vi "DataSender.vi"() -> ()   [LabVIEW 2013]
uses:
  <vilib>/userdefined/High Color/IMAQdx.ctl
  <vilib>/DAQmx/read.llb/DAQmx Read (Analog 2D DBL NChan NSamp).vi
  <vilib>/DAQmx/miscellaneous.llb/DAQmx Fill In Error Info.vi
  <vilib>/vision/driver/NI_Vision_Acquisition_Software.lvlib
panel:
  in  "Remote Host":string
  in  "Broadcast":bool
  in  "Remote Port":u16
  in  "Local Port":u16
  in  "stop 4":bool
  in  "stop 3":bool
  in  "stop 2":bool
  in  "BIN ON/OFF":bool
  in  "AVI ON/OFF":bool
  out "Frame number recorded":i32
  in  "Path":path
  in  "File number":i32
  out "error out":errorcluster
  in  "stop":bool
  out "image":T1(plugin-control)
  in  "Session In":T2
  # "M:\\Documents\\Master\\2.Semester\\FYS4240\\fys4240\\Lab4\\fys4240_lab4\\Lab4\\Videos"
  # "NOTE:"
  # "Remote Host:"
  # "Local Port: 61556"
  # "Remote Port: 61557"
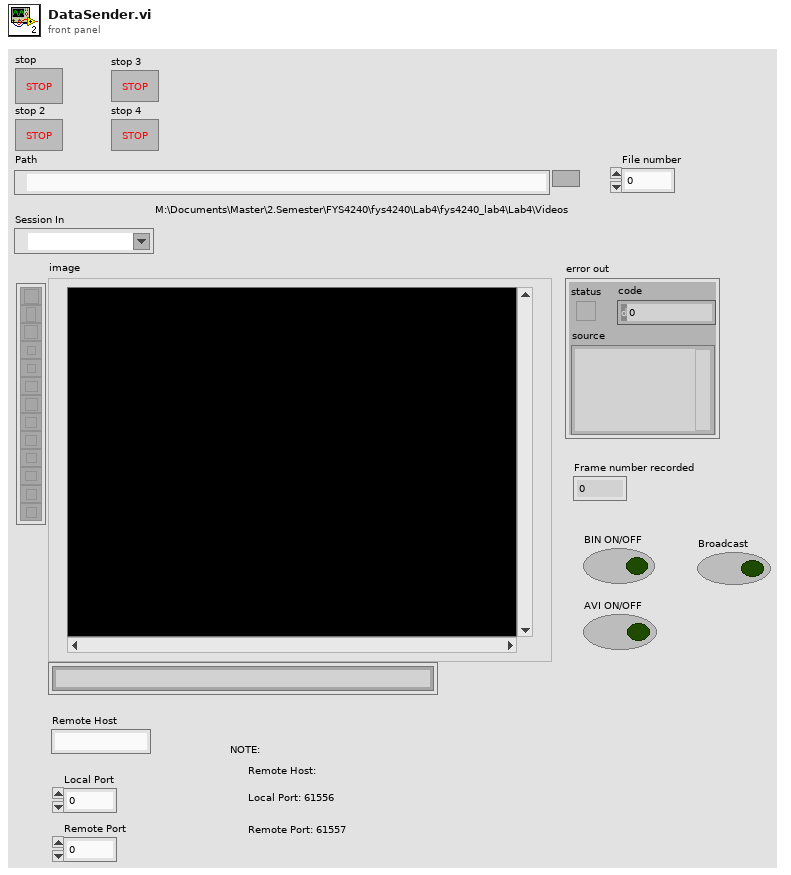
[diagram p1: front panel]
types:
  T1 = typedef "IMAQ Image.ctl" = refnum<image>
  T2 = typedef "IMAQdx.ctl" = refnum<k21>
  T3 = enum16{"big-endian, network order", "native, host order", "little-endian"}
  T4 = enum16{"open", "open or create", "create or replace", "create", "open (read-only)"}
  T5 = enum16{"open", "replace", "create", "open or create", "replace or create", "replace or create with confirmation"}
  T6 = typedef "Image Type" = u32
  T7 = typedef "IMAQ AVI2 Refnum.ctl" = refnum<k20>
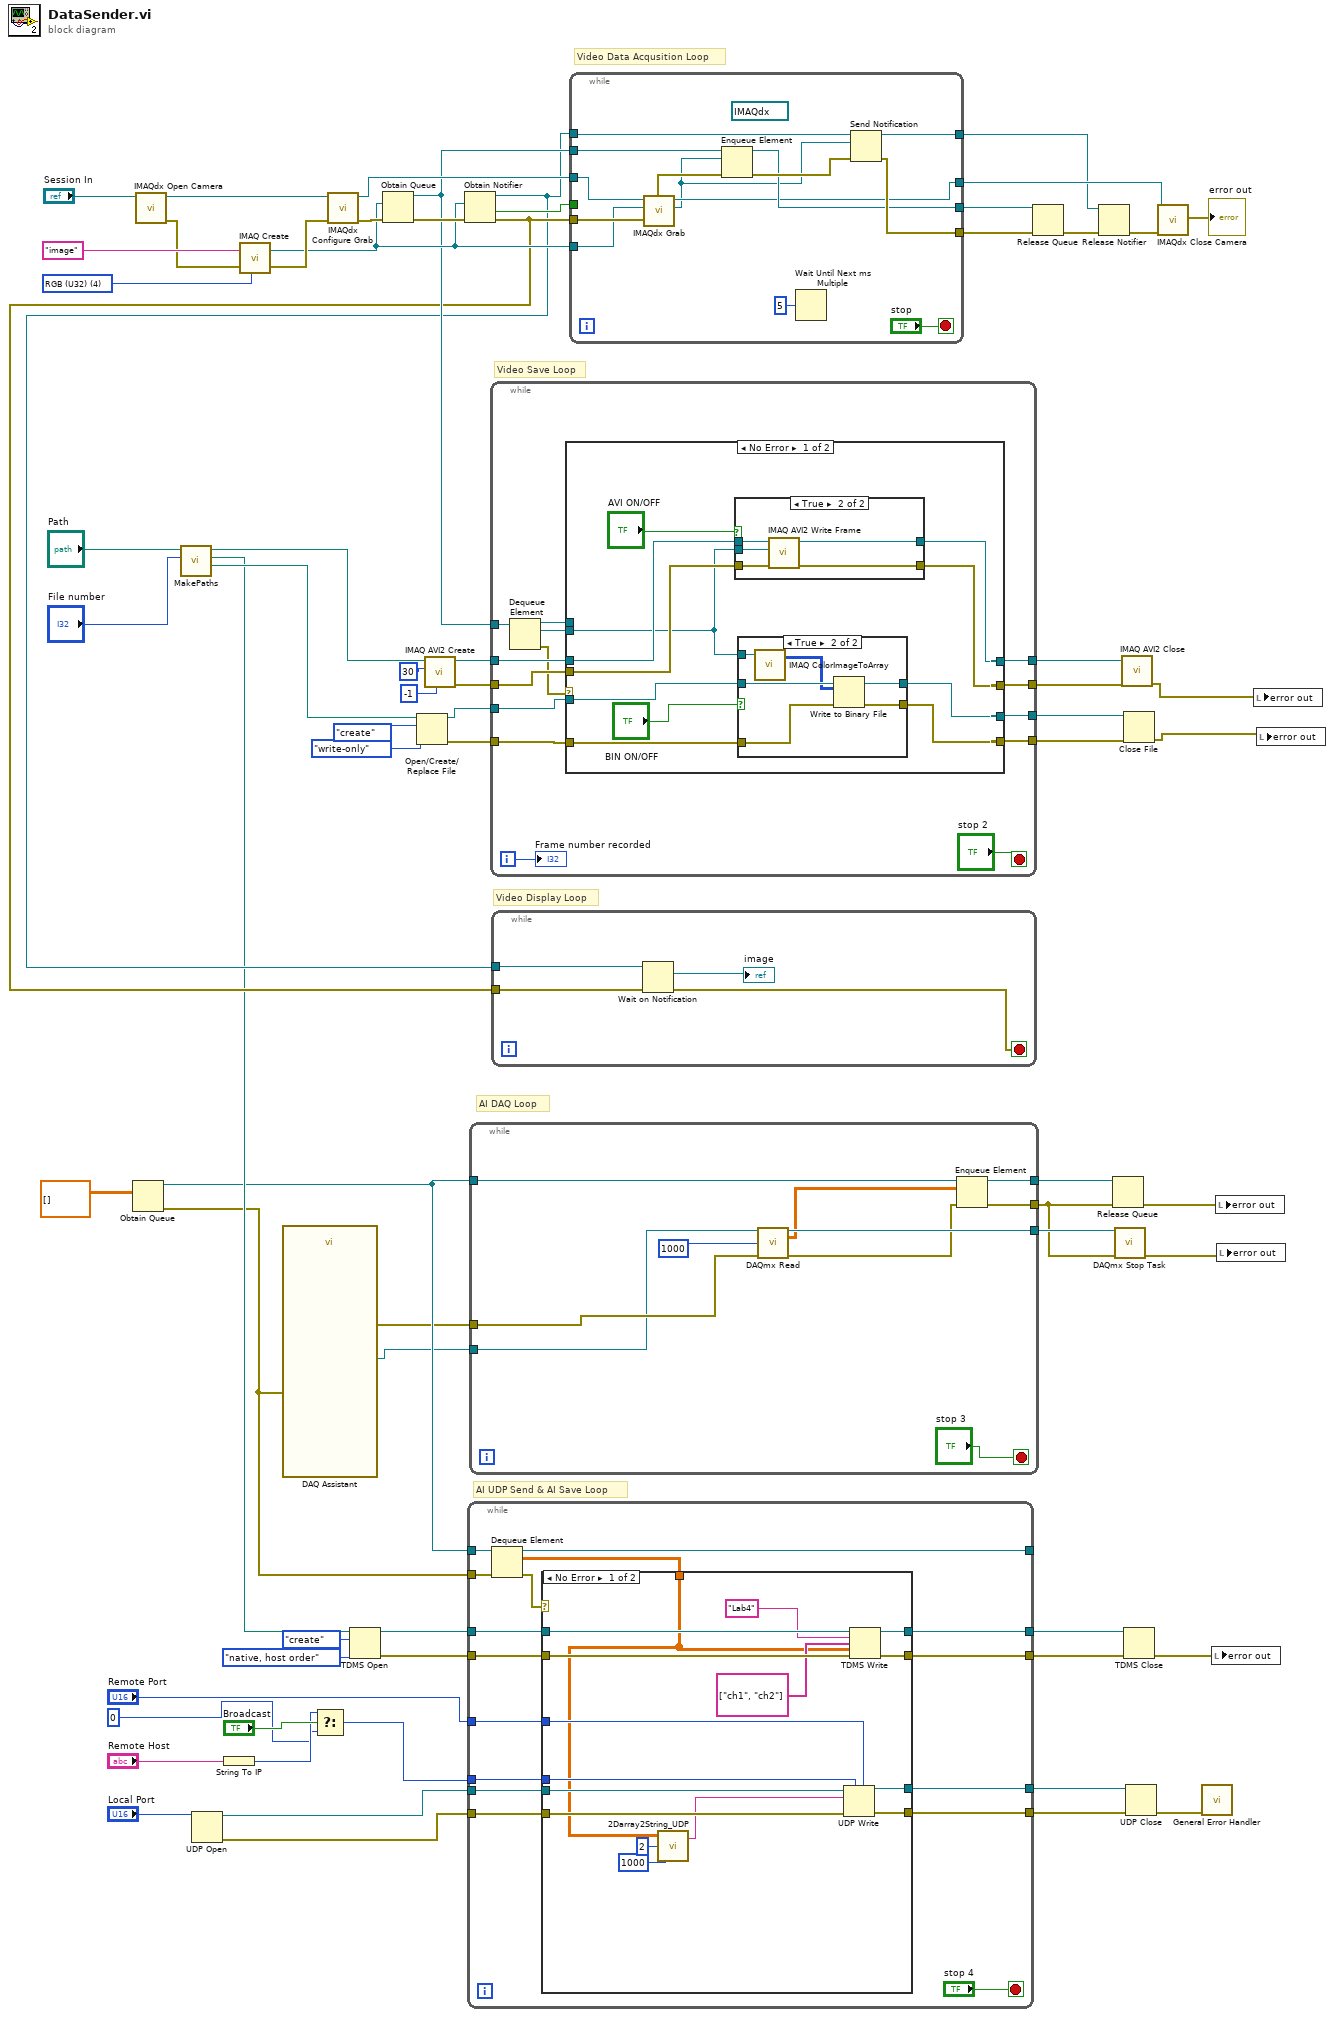
[diagram p0: block diagram]
diagram:
  w67 = T6 4 items=["Grayscale (U8)", "Grayscale (I16)", "Grayscale (SGL)", "Complex (CSG)", "RGB (U32)", "HSL (U32)", "RGB (U64)", "Grayscale (U16)"] ("Image Type")
  # "AI UDP Send & AI Save Loop"
  # "AI DAQ Loop"
  # "Video Data Acqusition Loop"
  # "Video Save Loop"
  # "Video Display Loop"
  n1 = Obtain Queue(element data type=dbl[][] []) -> (queue out=w20:refnum<queue>, error out=w14:errorcluster)  [unwired: 4 in, 1 out]
  n2 = call <vilib>:"IMAQdx Open Camera.vi"("Session In"="Session In") -> ("error out"=w66:errorcluster, "Session Out"=w65:T2)  [unwired: 9 in]
  n3 = call "MakePaths.vi"("number"="File number", "Path"="Path") -> ("BIN"=w40:path, "TDMS"=w21:path, "AVI"=w48:path)  [unwired: 7 in]
  n4 = UDP Open(11:"Local Port") -> (port=w6:refnum<k16>, 0:w3:errorcluster)  [unwired: 4 in, 1 out]
  n5 = String To IP(1:"Remote Host") -> (0:w2:u32)
  n6 = call "IMAQ Create"("Image Name"="image", "Image Type"=w67, "error in (no error)"=w66) -> ("New Image"=w52:T1, "error out"=w62:errorcluster)  [unwired: 2 in]
  n7 = call "DAQ Assistant"("error in"=w14) -> ("task out"=w7:refnum<k21>, "error out"=w15:errorcluster)  [unwired: 15 in, 2 out]
  n8 = Select(t=w2, s="Broadcast", f=u32 0 ("t")) -> (s? t:f=w4:u32)
  n9 = call <vilib>:"IMAQdx Configure Grab.vi"("error in"=w62, "Session In"=w65) -> ("error out"=w61:errorcluster, "Session Out"=w60:T2)  [unwired: 8 in]
  n10 = TDMS Open(9:T3."native, host order" ("byte order (2:little-endian)"), 10:T4."create" ("operation (0:open)"), 11:w21) -> (0:w25:errorcluster, 3:w22:refnum<k34>)  [unwired: 4 in]
  n11 = Obtain Queue(element data type=w52, error in (no error)=w61) -> (queue out=w35:refnum<queue>, error out=w64:errorcluster)  [unwired: 3 in, 1 out]
  n12 = Open/Create/Replace File(file path (use dialog)=w40, operation (0:open)=T5."create", access (0:read/write)=enum16{"read/write", "read-only", "write-only"}."write-only") -> (refnum out=w39:refnum<file>, error out=w41:errorcluster)  [unwired: 3 in, 1 out]
  n13 = call "IMAQ AVI2 Create"("Quality"=-1, "Frames Per Second"=u32 30, "AVI Path"=w48) -> ("error out"=w49:errorcluster, "AVI Refnum"=w47:T7)  [unwired: 7 in]
  n14 = Obtain Notifier(notification data type=w52, error in (no error)=w64) -> (notifier out=w31:refnum<notifier>, created new?=w53:bool, error out=w32:errorcluster)  [unwired: 2 in]
  n15 = while {
    tunnel: w25 -> [w82]
    tunnel: [w78] -> w24
    tunnel: [w79] -> w23
    tunnel: w22 -> [w81]
    tunnel: w14 -> [w85]
    tunnel: w20 -> [w84]
    tunnel: [w77] -> _
    tunnel: [w75] -> w9
    tunnel: [w74] -> w8
    tunnel: w3 -> [w73]
    tunnel: w6 -> [w72]
    tunnel: "Remote Port" -> [w71]
    tunnel: w4 -> [w70]
    stop <- "stop 4" stop-if-true
    n16 = Dequeue Element(queue=w84, error in (no error)=w85) -> (queue out=w77:refnum<queue>, element=w80:dbl[][], error out=w76:errorcluster)  [unwired: 1 in, 1 out]
    n17 = case shown="No Error" w76 {
      tunnel: w82 -> [w101 w105]
      tunnel: w81 -> [w100 w104]
      tunnel: w80 -> [w89 _]
      tunnel: [w99 w104] -> w79
      tunnel: [w98 w105] -> w78
      tunnel: [w94 w102] -> w75
      tunnel: [w95 w103] -> w74
      tunnel: w73 -> [w93 w103]
      tunnel: w72 -> [w92 w102]
      tunnel: w71 -> [w91 _]
      tunnel: w70 -> [w90 _]
      frame No Error {
        n18 = call "2Darray2String_UDP.vi"("NumOfCH"=1000, "NumberOfSamples"=2, "Waveform Graph"=w89) -> ("UDP_String"=w86:string)  [unwired: 1 out]
        n19 = UDP Write(address=w90, port or service name=w91, connection ID=w92, data in=w86, 8:w93) -> (error out=w95:errorcluster, 3:w94:refnum<k16>)  [unwired: 1 in]
        n20 = TDMS Write(0:w100, 5:"Lab4" ("group name in (Untitled)"), 7:string[] ["ch1", "ch2"] ("channel name(s) in (Untitled)"), 9:w89, 11:w101) -> (4:w99:refnum<k34>, 15:w98:errorcluster)  [unwired: 1 in, 2 out]
      }
      frame Error {
      }
    }
  }
  n21 = while {
    tunnel: w20 -> [w115]
    tunnel: [w114] -> w30
    tunnel: [w113] -> w16
    tunnel: [w112] -> w29
    tunnel: w15 -> [w107]
    tunnel: w7 -> [w106]
    stop <- "stop 3" stop-if-true
    n22 = call-poly <vilib>:"DAQmx Read.vi"("task/channels in"=w106, "number of samples per channel"=1000, "error in"=w107) -> ("task out"=w112:refnum<k21>, "data"=w111:dbl[][], "error out"=w108:errorcluster)  [unwired: 10 in]
    n23 = Enqueue Element(queue=w115, element=w111, error in (no error)=w108) -> (queue out=w114:refnum<queue>, error out=w113:errorcluster)  [unwired: 1 in, 1 out]
  }
  n24 = while {
    tunnel: [w129] -> w50
    tunnel: w49 -> [w127]
    tunnel: w47 -> [w126]
    tunnel: [w125] -> w46
    tunnel: w35 -> [w124]
    tunnel: [w120] -> w42
    tunnel: w41 -> [w119]
    tunnel: w39 -> [w118]
    tunnel: [w117] -> w38
    i -> [w128]
    stop <- "stop 2" stop-if-true
    n25 = Dequeue Element(queue=w124) -> (queue out=w123:refnum<queue>, element=w121:T1, error out=w122:errorcluster)  [unwired: 2 in, 1 out]
    n26 = case shown="No Error" w122 {
      tunnel: [w132 w158] -> w129
      tunnel: w127 -> [w140 w158]
      tunnel: w126 -> [w139 w159]
      tunnel: [w138 w159] -> w125
      tunnel: w123 -> [_ _]
      tunnel: w121 -> [w134 _]
      tunnel: [w137 w157] -> w120
      tunnel: w119 -> [w136 w157]
      tunnel: w118 -> [w135 w156]
      tunnel: [w133 w156] -> w117
      frame No Error {
        n27 = case shown="True" "AVI ON/OFF" {
          tunnel: [w149 w155] -> w132
          tunnel: w140 -> [w149 w154]
          tunnel: w139 -> [w150 w153]
          tunnel: [w150 w152] -> w138
          tunnel: w134 -> [_ w151]
          frame False {
          }
          frame True {
            n28 = call "IMAQ AVI2 Write Frame"("error in (no error)"=w154, "Image"=w151, "AVI Refnum"=w153) -> ("error out"=w155:errorcluster, "AVI Refnum (duplicate)"=w152:T7)  [unwired: 6 in, 1 out]
          }
        }
        n29 = case shown="True" "BIN ON/OFF" {
          tunnel: [w141 w148] -> w137
          tunnel: w136 -> [w141 w147]
          tunnel: w135 -> [w142 w146]
          tunnel: w134 -> [_ w144]
          tunnel: [w142 w143] -> w133
          frame False {
          }
          frame True {
            n30 = call "IMAQ ColorImageToArray"("Image"=w144) -> ("Image Pixels (U32)"=w145:u32[][])  [unwired: 3 in, 2 out]
            n31 = Write to Binary File(file (use dialog)=w146, data=w145, error in=w147) -> (refnum out=w143:refnum<file>, error out=w148:errorcluster)  [unwired: 3 in, 1 out]
          }
        }
      }
      frame Error {
      }
    }
    "Frame number recorded" <- w128
  }
  n32 = while {
    tunnel: w32 -> [w163]
    tunnel: w31 -> [w162]
    stop <- w160 stop-if-true
    n33 = Wait on Notification(notifier=w162, error in (no error)=w163) -> (notification=→"image":T1, error out=w160:errorcluster)  [unwired: 2 in, 2 out]
  }
  n34 = while {
    tunnel: [w165] -> w57
    tunnel: w32 -> [w175]
    tunnel: w60 -> [w166]
    tunnel: [w174] -> w56
    tunnel: [w173] -> w55
    tunnel: w35 -> [w170]
    tunnel: [w169] -> w54
    tunnel: w52 -> [w168]
    tunnel: w31 -> [w167]
    tunnel: w53 -> [_]
    stop <- "stop" stop-if-true
    (unwired) T2 "cam0" ("notification")
    n35 = call <vilib>:"IMAQdx Grab.vi"("error in"=w175, "Image In"=w168, "Session In"=w166) -> ("error out"=w172:errorcluster, "Image Out"=w164:T1, "Session Out"=w165:T2)  [unwired: 5 in, 1 out]
    n36 = Enqueue Element(queue=w170, element=w164, error in (no error)=w172) -> (queue out=w169:refnum<queue>, error out=w171:errorcluster)  [unwired: 1 in, 1 out]
    n37 = Wait Until Next ms Multiple(millisecond multiple=u32 5) -> ()  [unwired: 1 out]
    n38 = Send Notification(notification=w164, notifier=w167, error in (no error)=w171) -> (notifier out=w174:refnum<notifier>, error out=w173:errorcluster)
  }
  n39 = Release Queue(queue=w54, error in (no error)=w55) -> (error out=w59:errorcluster)  [unwired: 1 in, 2 out]
  n40 = Release Notifier(notifier=w56, error in (no error)=w59) -> (error out=w58:errorcluster)  [unwired: 1 in, 2 out]
  n41 = Release Queue(queue=w30, error in (no error)=w16) -> (error out=w28:errorcluster)  [unwired: 1 in, 2 out]
  n42 = call <vilib>:"DAQmx Stop Task.vi"("task/channels in"=w29, "error in"=w16) -> ("error out"=w27:errorcluster)  [unwired: 12 in, 1 out]
  n43 = call "IMAQ AVI2 Close"("error in (no error)"=w50, "AVI Refnum"=w46) -> ("error out"=w34:errorcluster)  [unwired: 9 in]
  n44 = Close File(refnum=w38, error in=w42) -> (error out=w33:errorcluster)  [unwired: 1 out]
  n45 = TDMS Close(8:w24, 11:w23) -> (0:w17:errorcluster)  [unwired: 1 out]
  n46 = UDP Close(connection ID=w9, 8:w8) -> (error out=w10:errorcluster)  [unwired: 1 out]
  n47 = call <vilib>:"IMAQdx Close Camera.vi"("error in"=w58, "Session In"=w57) -> ("error out"=→"error out":errorcluster)  [unwired: 9 in]
  n48 = call <vilib>:"General Error Handler.vi"("error in (no error)"=w10) -> ()  [unwired: 10 in, 5 out]
  n49 = local write "error out"(w17) -> ()
  n50 = local write "error out"(w28) -> ()
  n51 = local write "error out"(w27) -> ()
  n52 = local write "error out"(w34) -> ()
  n53 = local write "error out"(w33) -> ()
